vi "Write DCIMG.vi"(8 "error in (no error)":errorcluster, 10 "DCIMG":cluster{"File1":path, "File2":path}, 11 "Tiff Writer in":refnum<class "Tiff Writer.lvclass">) -> (0 "error out":errorcluster, 3 "Tiff Writer out":refnum<class "Tiff Writer.lvclass">)   [LabVIEW 2015, in "Tiff Writer.lvlib" / "Tiff Writer.lvclass"]
uses:
  Tiff Writer.lvclass
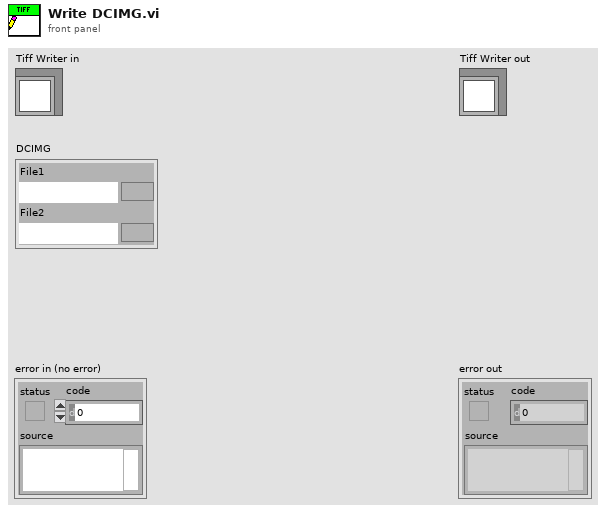
[diagram p1: front panel]
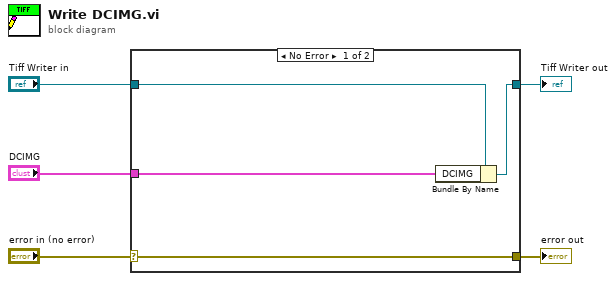
[diagram p0: block diagram]
diagram:
  n1 = case shown="No Error" "error in (no error)" {
    selector: "error in (no error)" -> [w9 w10]
    tunnel: [w9 w10] -> w4
    tunnel: [w7 w11] -> w2
    tunnel: "Tiff Writer in" -> [w8 w11]
    tunnel: "DCIMG" -> [w6 _]
    frame No Error {
      n2 = Bundle By Name(cluster=w8, "DCIMG"=w6) -> (w7:refnum<class "Tiff Writer.lvclass">)
    }
    frame Error {
    }
  }
  "error out" <- w4
  "Tiff Writer out" <- w2
